vi "Reset.vi"(8 "error in":errorcluster, 11 "VISA resource name in":refnum<visa-resource-name>) -> (0 "error out":errorcluster, 2 "Prompt":string, 3 "VISA resource name out":refnum<visa-resource-name>)   [LabVIEW 2021, in "Keysight U1282A.lvlib"]
doc: "El comando reset (*RST) coloca al U1281A/U1282A en el estado de power-on-reset sin apagar la línea de energía y regresa la posición actual del selector del multímetro ('Prompt\")."
uses:
  Keysight U1282A.lvlib
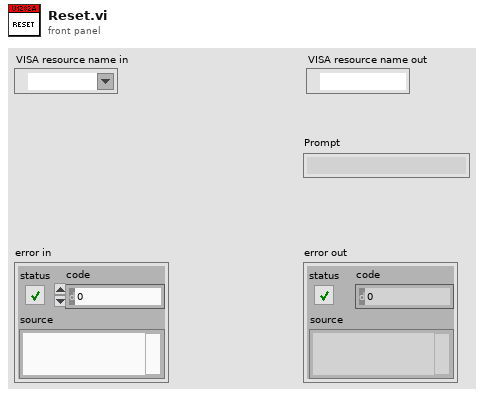
[diagram p1: front panel]
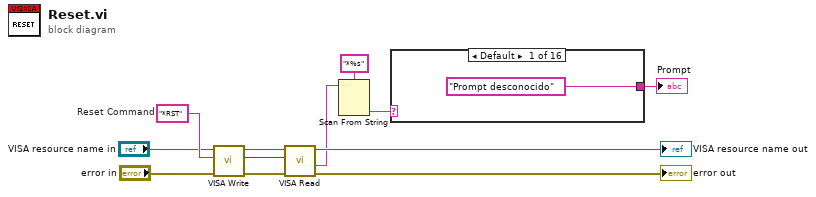
[diagram p0: block diagram]
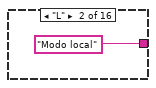
[diagram p2: hidden frame]
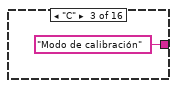
[diagram p3: hidden frame]
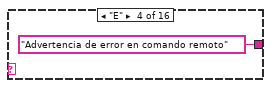
[diagram p4: hidden frame]
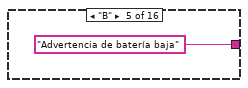
[diagram p5: hidden frame]
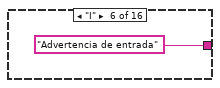
[diagram p6: hidden frame]
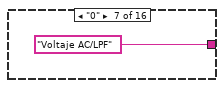
[diagram p7: hidden frame]
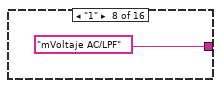
[diagram p8: hidden frame]
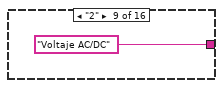
[diagram p9: hidden frame]
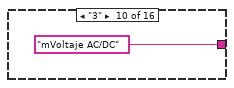
[diagram p10: hidden frame]
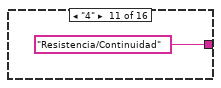
[diagram p11: hidden frame]
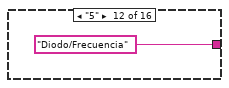
[diagram p12: hidden frame]
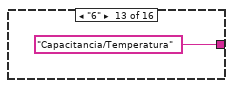
[diagram p13: hidden frame]
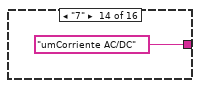
[diagram p14: hidden frame]
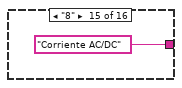
[diagram p15: hidden frame]
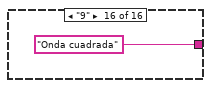
[diagram p16: hidden frame]
diagram:
  w8 = "*RST"  # Reset Command
  n1 = call "VISA Write.vi"("error in"="error in", "SCPI command"=w8, "VISA resource in"="VISA resource name in") -> ("error out"=w6:errorcluster, "Bytes at Port out"=w5:u32, "VISA resource out"=w4:refnum<visa-resource-name>)  [unwired: 6 in]
  n2 = call "VISA Read.vi"("error in"=w6, "Bytes at Port in"=w5, "VISA resource in"=w4) -> ("error out"=→"error out":errorcluster, "Reading"=w1:string, "VISA resource out"=→"VISA resource name out":refnum<visa-resource-name>)  [unwired: 5 in, 1 out]
  n3 = Scan From String(format string="*%s", input string=w1) -> (output 1=w11:string)  [unwired: 3 in, 3 out]
  n4 = case shown="Default" w11 {
    tunnel: ["Prompt desconocido" ("Prompt") "Modo local" ("Prompt") "Modo de calibración" ("Prompt") "Advertencia de error en comando remoto" ("Prompt") "Advertencia de batería baja" ("Prompt") "Advertencia de entrada" ("Prompt") "Voltaje AC/LPF" ("Prompt") "mVoltaje AC/LPF" ("Prompt") "Voltaje AC/DC" ("Prompt") "mVoltaje AC/DC" ("Prompt") "Resistencia/Continuidad" ("Prompt") "Diodo/Frecuencia" ("Prompt") "Capacitancia/Temperatura" ("Prompt") "umCorriente AC/DC" ("Prompt") "Corriente AC/DC" ("Prompt") "Onda cuadrada" ("Prompt")] -> w10
    frame Default {
    }
    frame "L" {
    }
    frame "C" {
    }
    frame "E" {
    }
    frame "B" {
    }
    frame "I" {
    }
    frame "0" {
    }
    frame "1" {
    }
    frame "2" {
    }
    frame "3" {
    }
    frame "4" {
    }
    frame "5" {
    }
    frame "6" {
    }
    frame "7" {
    }
    frame "8" {
    }
    frame "9" {
    }
  }
  "Prompt" <- w10
